vi "test Pic.vi"() -> ()   [LabVIEW 2018, in "Picture Process.lvclass"]
uses:
  Picture Process.lvclass
  <vilib>/picture/picture.llb/Draw True-Color Pixmap.vi
panel:
  in  "Color":u32(colorbox)=6618880
  in  "Line":cluster{"Size":i32, "Width":u16}={"Size"=3, "Width"=1}
  in  "Position":cluster{"Centerx":i32, "Centery":i32}
  in  "subset rect":T1
  out "2D Picture":picture
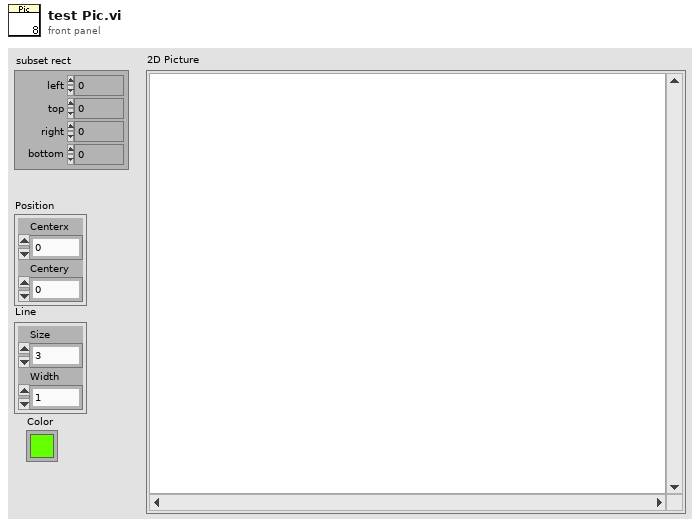
[diagram p1: front panel]
types:
  T1 = cluster{"left":i16, "top":i16, "right":i16, "bottom":i16}
  T2 = typedef "imagedata.ctl" = cluster{"image type":i32, "image depth":i32, "image":u8[], "mask":u8[], "colors":u32[], "Rectangle":cluster{"left":i16, "top":i16, "right":i16, "bottom":i16}}
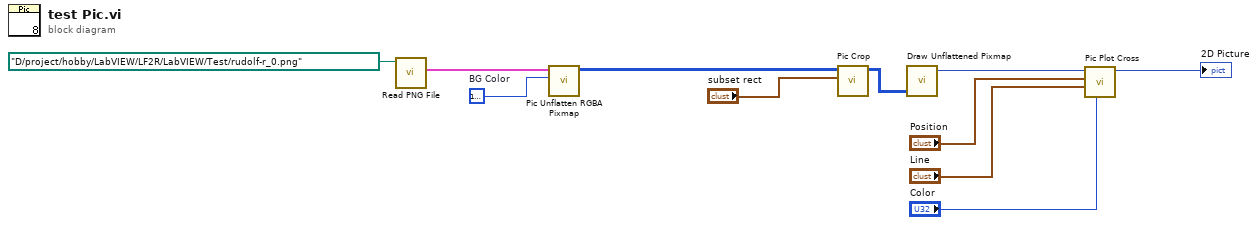
[diagram p0: block diagram]
diagram:
  w6 = u32 16777222  # BG Color
  n1 = call <vilib>:"Read PNG File.vi"("path to PNG file"=path "D:/project/hobby/LabVIEW/LF2R/LabVIEW/Test/rudolf-r_0.png") -> ("image data"=w8:T2)  [unwired: 8 in, 2 out]
  n2 = call "Pic Unflatten RGBA Pixmap.vi"("BG Color"=w6, "32-bit image data (ARGB)"=w8) -> ("24-bit pixmap"=w7:u32[][])  [unwired: 8 in, 1 out]
  n3 = call "Pic Crop.vi"("Position"="subset rect", "24-bit pixmap in"=w7) -> ("24-bit pixmap out"=w10:u32[][])  [unwired: 8 in, 1 out]
  n4 = call-poly <vilib>:"Draw Unflattened Pixmap.vi"("data (RGB format)"=w10) -> ("new picture"=w5:picture)  [unwired: 8 in]
  n5 = call "Pic Plot Cross.vi"("Color"="Color", "Line"="Line", "Position"="Position", "Picture in"=w5) -> ("Picture out"=→"2D Picture":picture)  [unwired: 6 in, 1 out]
